vi "Construct Listbox Bus Monitor.vi"(10 "Show Panel Boolean Name":string) -> (3 "ListboxBusMonitor out":refnum<class "ListboxBusMonitor.lvclass">)   [LabVIEW 2020, in "MVA Framework.lvlib" / "ListboxBusMonitor.lvlib" / "ListboxBusMonitor.lvclass"]
doc: "构建列表框总线监视器"
uses:
  ListboxBusMonitor.lvclass
  ListboxBusMonitor.lvclass/ListboxBusMonitor.ctl
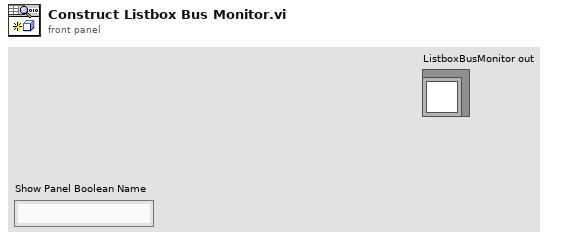
[diagram p1: front panel]
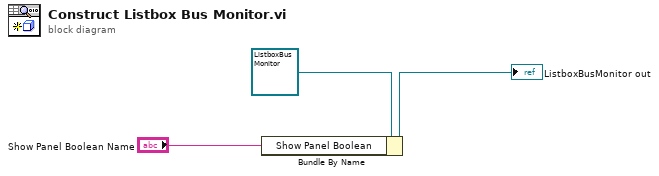
[diagram p0: block diagram]
diagram:
  n1 = Bundle By Name(cluster=refnum<class "ListboxBusMonitor.lvclass"> refnum ("ListboxBusMonitor in"), "Show Panel Boolean"="Show Panel Boolean Name") -> (→"ListboxBusMonitor out":refnum<class "ListboxBusMonitor.lvclass">)
